vi "calcula_dora.vi"   [LabVIEW 2020]
uses:
  GlobalVariables.vi
  <vilib>/Rock Robotics/Network Tables/NT Read Number.vi
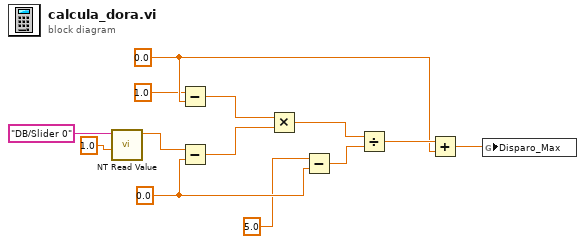
[diagram p0: block diagram]
diagram:
  w5 = 0.0 ("y")
  w6 = 0.0 ("y")
  n1 = call-poly <vilib>:"NT Read Value.vi"("Default Value"=1.0, "Name"="DB/Slider 0" ("refnum name")) -> ("Numeric"=w1:dbl)  [unwired: 8 in, 1 out]
  n2 = Subtract(x=1.0, y=w6) -> (x-y=w7:dbl)
  n3 = Subtract(x=w1, y=w5) -> (x-y=w8:dbl)
  n4 = Multiply(x=w7, y=w8) -> (x*y=w9:dbl)
  n5 = Subtract(x=5.0, y=w5) -> (x-y=w10:dbl)
  n6 = Divide(x=w9, y=w10) -> (x/y=w11:dbl)
  n7 = Add(x=w11, y=w6) -> (x+y=w2:dbl)
  n8 = global write "GlobalVariables.vi" "Disparo_Max"(w2) -> ()
